vi "PRAT Read All MW100 Inputs.vi"(0 "MW100":refnum<visa-resource-name>="MW100", 11 "Error In":errorcluster) -> (4 "dup VISA session":refnum<visa-resource-name>, 6 "PowerData":T1, 15 "error out":errorcluster)   [LabVIEW 2016]
uses:
  Type Definitions/HEWH Power Data.ctl
  Type Definitions/PRAT Channel Settings.ctl
panel:
  out "Channel List":string[](array[string])
  out "All Data":dbl[](array[numeric]) format="%.4f"
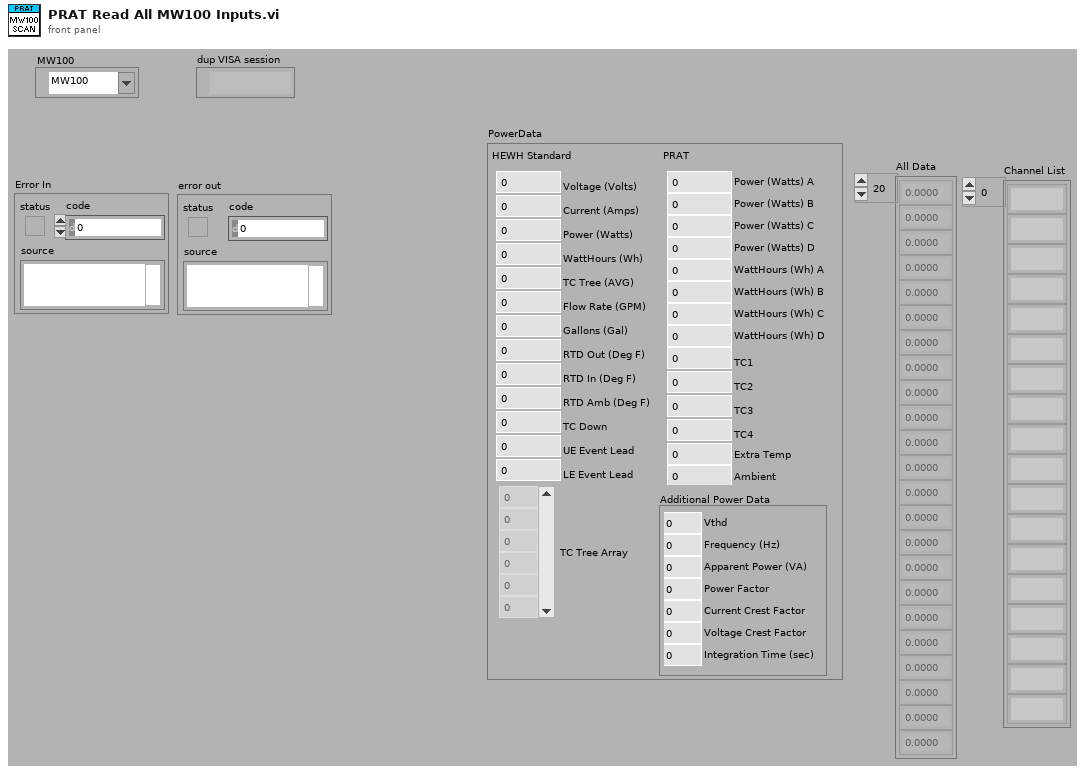
[diagram p1: front panel]
types:
  T1 = typedef "HEWH Power Data.ctl" = cluster{"HEWH Standard":cluster{"Voltage (Volts)":dbl, "Current (Amps)":dbl, "Power (Watts)":dbl, "WattHours (Wh)":dbl, "TC Tree (AVG)":dbl, "Flow Rate (GPM)":dbl, "Gallons (Gal)":dbl, "RTD Out (Deg F)":dbl, "RTD In (Deg F)":dbl, "RTD Amb (Deg F)":dbl, "TC Down":dbl, "UE Event Lead":i32, "LE Event Lead":i32, "TC Tree Array":dbl[]}, "PRAT":cluster{"Power (Watts) A":dbl, "Power (Watts) B":dbl, "Power (Watts) C":dbl, "Power (Watts) D":dbl, "TC1":dbl, "TC2":dbl, "TC3":dbl, "TC4":dbl, "WattHours (Wh) A":dbl, "WattHours (Wh) B":dbl, "WattHours (Wh) C":dbl, "WattHours (Wh) D":dbl, "Ambient":dbl, "Extra Temp":dbl}, "Additional Power Data":cluster{"Vthd":dbl, "Frequency (Hz)":dbl, "Apparent Power (VA)":dbl, "Power Factor":dbl, "Current Crest Factor":dbl, "Voltage Crest Factor":dbl, "Integration Time (sec)":dbl}}
  T2 = typedef "PRAT Channel Settings.ctl" = string
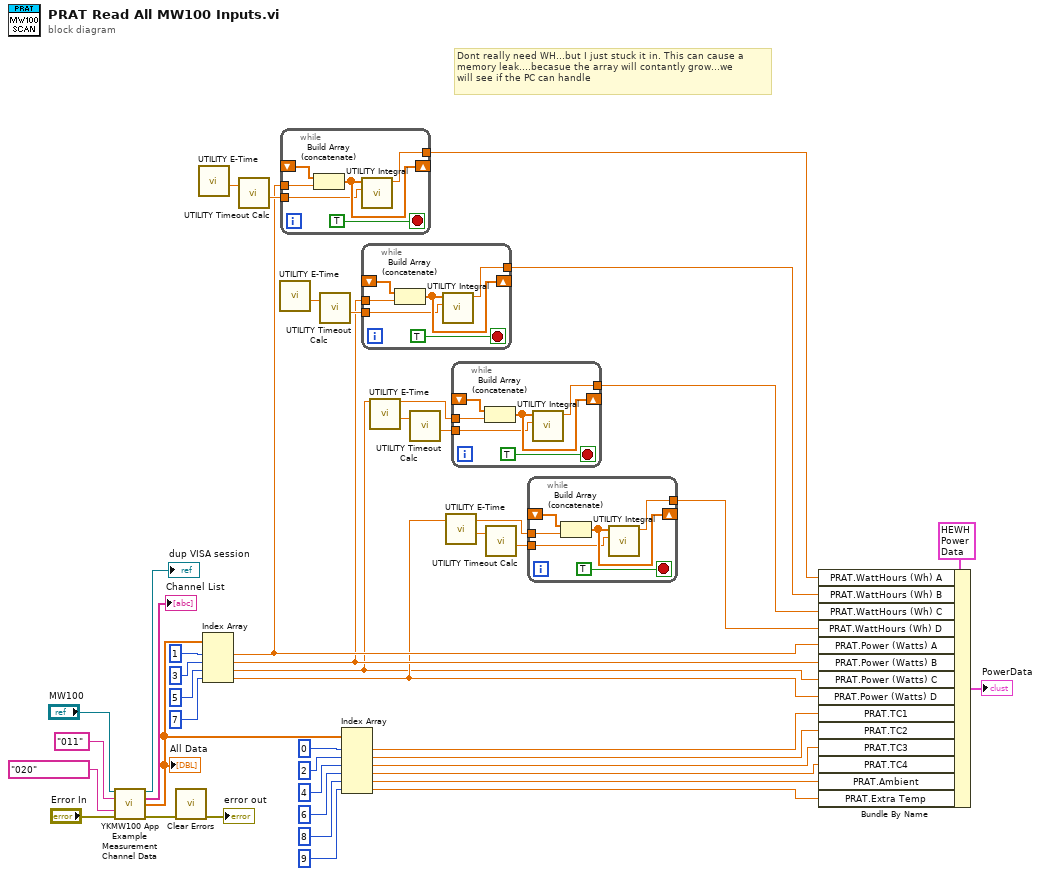
[diagram p0: block diagram]
diagram:
  # "Dont really need WH...but I just stuck it in. This can cause a \nmemory leak....becasue the array will contantly grow...we \nwill see if the PC can handle"
  n1 = call "YKMW100 App Example Measurement Channel Data.vi"("VISA session"="MW100", "Start Channel (001)"=T2 "011" ("PRAT Channels"), "End Channel (001)"=T2 "020" ("PRAT Channels"), "error in (no error)"="Error In") -> ("dup VISA session"=→"dup VISA session":refnum<visa-resource-name>, "Channel List"=→"Channel List":string[], "Data List"=w26:dbl[], "error out"=w18:errorcluster)  [unwired: 4 in, 4 out]
  "All Data" <- w26
  n2 = call <vilib>:"Clear Errors.vi"("error in (no error)"=w18) -> ("error out"=→"error out":errorcluster)  [unwired: 5 in, 1 out]
  n3 = call "UTILITY E-Time.vi"() -> ("Elapsed Time (sec)"=w16:dbl)  [unwired: 9 in, 2 out]
  n4 = Index Array(array=w26, index #1=1 ("index"), index #2=3 ("index"), index #3=5 ("index"), index #4=7 ("index")) -> (element #1=w14:dbl, element #2=w10:dbl, element #3=w3:dbl, element #4=w4:dbl)
  n5 = call "UTILITY Timeout Calc.vi"("Timer"=w16) -> ("Rate"=w15:dbl)  [unwired: 9 in, 1 out]
  n6 = call "UTILITY E-Time.vi"() -> ("Elapsed Time (sec)"=w11:dbl)  [unwired: 9 in, 2 out]
  n7 = while {
    shift-right: [w48] -> _
    shift-left: _ -> [w49]
    tunnel: w15 -> [w47]
    tunnel: [w46] -> w13
    tunnel: w14 -> [w45]
    stop <- TRUE stop-if-true
    n8 = Build Array (concatenate)(w49, w45) -> (w48:dbl[])
    n9 = call "UTILITY Integral.vi"("dt"=w47, "Array Input"=w48) -> ("Integral"=w46:dbl)  [unwired: 8 in, 1 out]
  }
  n10 = call "UTILITY Timeout Calc.vi"("Timer"=w11) -> ("Rate"=w12:dbl)  [unwired: 9 in, 1 out]
  n11 = Index Array(array=w26, index #1=0 ("index"), index #2=2 ("index"), index #3=4 ("index"), index #4=6 ("index"), index #5=8 ("index"), index #6=9 ("index")) -> (element #1=w36:dbl, element #2=w35:dbl, element #3=w34:dbl, element #4=w33:dbl, element #5=w20:dbl, element #6=w19:dbl)
  n12 = while {
    shift-right: [w54] -> _
    shift-left: _ -> [w55]
    tunnel: w12 -> [w53]
    tunnel: [w52] -> w9
    tunnel: w10 -> [w51]
    stop <- TRUE stop-if-true
    n13 = Build Array (concatenate)(w55, w51) -> (w54:dbl[])
    n14 = call "UTILITY Integral.vi"("dt"=w53, "Array Input"=w54) -> ("Integral"=w52:dbl)  [unwired: 8 in, 1 out]
  }
  n15 = call "UTILITY E-Time.vi"() -> ("Elapsed Time (sec)"=w8:dbl)  [unwired: 9 in, 2 out]
  n16 = call "UTILITY Timeout Calc.vi"("Timer"=w8) -> ("Rate"=w7:dbl)  [unwired: 9 in, 1 out]
  n17 = call "UTILITY E-Time.vi"() -> ("Elapsed Time (sec)"=w5:dbl)  [unwired: 9 in, 2 out]
  n18 = while {
    shift-right: [w60] -> _
    shift-left: _ -> [w61]
    tunnel: w7 -> [w59]
    tunnel: [w58] -> w2
    tunnel: w3 -> [w57]
    stop <- TRUE stop-if-true
    n19 = Build Array (concatenate)(w61, w57) -> (w60:dbl[])
    n20 = call "UTILITY Integral.vi"("dt"=w59, "Array Input"=w60) -> ("Integral"=w58:dbl)  [unwired: 8 in, 1 out]
  }
  n21 = call "UTILITY Timeout Calc.vi"("Timer"=w5) -> ("Rate"=w6:dbl)  [unwired: 9 in, 1 out]
  n22 = while {
    shift-right: [w66] -> _
    shift-left: _ -> [w67]
    tunnel: w6 -> [w65]
    tunnel: [w64] -> w1
    tunnel: w4 -> [w63]
    stop <- TRUE stop-if-true
    n23 = Build Array (concatenate)(w67, w63) -> (w66:dbl[])
    n24 = call "UTILITY Integral.vi"("dt"=w65, "Array Input"=w66) -> ("Integral"=w64:dbl)  [unwired: 8 in, 1 out]
  }
  n25 = Bundle By Name(cluster=T1 {"HEWH Standard"={"Voltage (Volts)"=240.0, "Current (Amps)"=0.017575, "Power (Watts)"=4.218, "WattHours (Wh)"=19682.0, "TC Tree (AVG)"=0.0, "Flow Rate (GPM)"=0.0, "Gallons (Gal)"=0.0, "RTD Out (Deg F)"=0.0, "RTD In (Deg F)"=0.0, "RTD Amb (Deg F)"=0.0, "TC Down"=0.0, "UE Event Lead"=0, "LE Event Lead"=0, "TC Tree Array"=[]}, "PRAT"={"Power (Watts) A"=4192.0, "Power (Watts) B"=4192.0, "Power (Watts) C"=4192.0, "Power (Watts) D"=4192.0, "TC1"=0.0, "TC2"=0.0, "TC3"=0.0, "TC4"=0.0, "WattHours (Wh) A"=4192.0, "WattHours (Wh) B"=4192.0, "WattHours (Wh) C"=4192.0, "WattHours (Wh) D"=4192.0, "Ambient"=0.0, "Extra Temp"=0.0}, "Additional Power Data"={"Vthd"=236.2, "Frequency (Hz)"=236.2, "Apparent Power (VA)"=236.2, "Power Factor"=236.2, "Current Crest Factor"=236.2, "Voltage Crest Factor"=236.2, "Integration Time (sec)"=236.2}} ("PowerData 2"), "PRAT.WattHours (Wh) A"=w13, "PRAT.WattHours (Wh) B"=w9, "PRAT.WattHours (Wh) C"=w2, "PRAT.WattHours (Wh) D"=w1, "PRAT.Power (Watts) A"=w14, "PRAT.Power (Watts) B"=w10, "PRAT.Power (Watts) C"=w3, "PRAT.Power (Watts) D"=w4, "PRAT.TC1"=w36, "PRAT.TC2"=w35, "PRAT.TC3"=w34, "PRAT.TC4"=w33, "PRAT.Ambient"=w20, "PRAT.Extra Temp"=w19) -> (→"PowerData":T1)
